vi "CheckForMenu.vi"(7 "Restart? (F)":bool, 8 "error in (no error)":errorcluster, 11 "Snake in":refnum<class "Game.lvclass">) -> (0 "error out":errorcluster, 2 "Restart out":bool, 3 "Snake out":refnum<class "Game.lvclass">)   [LabVIEW 2019, in "RT_Game.lvlib" / "Game.lvclass"]
uses:
  Game.lvclass
  Game.lvclass/Game.ctl
  MainMenu/MainMenu.lvclass
  C:/Users/FreshBob/Dropbox/VIs/myRIO_GameConsole/RT/RT_Game/Game/Game.lvclass
  Write SwitchGame.vi
  Write FlattenedNextClass.vi
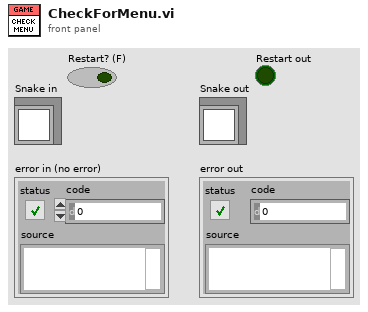
[diagram p1: front panel]
types:
  T1 = cluster{"Controls_1":cluster{"DirectionX":i8, "DirectionY":i8, "Button1":bool, "Button2":bool}, "Controls_2":cluster{"DirectionX":i8, "DirectionY":i8, "Button1":bool, "Button2":bool}, "SystemButton":bool}
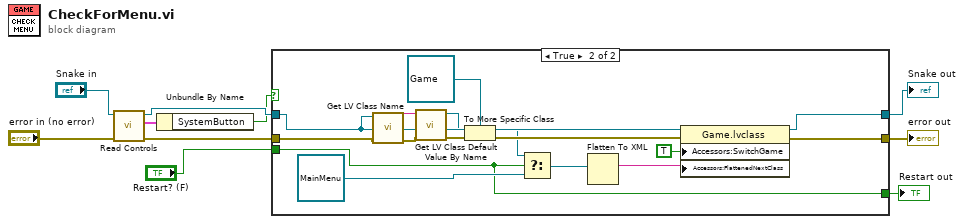
[diagram p0: block diagram]
diagram:
  n1 = call "Read Controls.vi"("error in (no error)"="error in (no error)", "Game in"="Snake in") -> ("error out"=w7:errorcluster, "Controls"=w4:T1, "Game out"=w5:refnum<class "Game.lvclass">)  [unwired: 7 in]
  n2 = Unbundle By Name(w4) -> ("SystemButton"=w3:bool)
  n3 = case shown="True" w3 {
    tunnel: [w11 w28] -> w9
    tunnel: w5 -> [w12 w22]
    tunnel: [w12 w27] -> w8
    tunnel: w7 -> [w11 w21]
    tunnel: "Restart? (F)" -> [_ w13]
    tunnel: [_ w13] -> w1
    frame False {
    }
    frame True {
      n4 = call <vilib>:"Get LV Class Name.vi"("error in (no error)"=w21, "object"=w22) -> ("error out"=w20:errorcluster, "class name"=w18:string)  [unwired: 8 in]
      n5 = call <vilib>:"Get LV Class Default Value By Name.vi"("error in (no error)"=w20, "class name"=w18) -> ("error out"=w19:errorcluster, "object"=w16:refnum<class>)  [unwired: 8 in]
      n6 = To More Specific Class(target class=refnum<class "Game.lvclass"> refnum ("Game out"), reference=w16, error in=w19) -> (specific class reference=w14:refnum<class "Game.lvclass">, error out=w17:errorcluster)
      n7 = Select(t=w14, s=w13, f=refnum<class "MainMenu.lvclass"> refnum ("RT_Game.lvlib:MainMenu.lvclass")) -> (s? t:f=w24:refnum<class "Game.lvclass">)
      n8 = Flatten To XML(anything=w24) -> (xml string=w25:string)
      n9 = property class="Game.lvclass"(reference=w22, error in=w17, "Accessors:SwitchGame"=TRUE ("SwitchGame_"), "Accessors:FlattenedNextClass"=w25) -> (reference out=w27:refnum<class "Game.lvclass">, error out=w28:errorcluster)
    }
  }
  "Snake out" <- w8
  "error out" <- w9
  "Restart out" <- w1
